vi "RenameEventNames.vi"(8 "Write":refnum<user-event>[](array[refnum]), 9 "Read":refnum<user-event>[](array[refnum]), 10 "State":refnum<user-event>[](array[refnum]), 11 "Error":refnum<user-event>[](array[refnum])) -> (0 "Write":refnum<user-event>[](array[refnum]), 1 "Read":refnum<user-event>[](array[refnum]), 2 "State":refnum<user-event>[](array[refnum]), 3 "Error":refnum<user-event>[](array[refnum]))   [LabVIEW 2016, in "lockin.lvclass"]
uses:
  lockin.lvclass
  DAQ/Typedefs/PublicEvents--DAQ.Read.ctl
  <vilib>/JKI/JKI SMO/SMO/Typedefs/SMOState --Enum.ctl
  DAQ/Typedefs/PublicEvents--DAQ.Write.ctl
  DAQ/DAQ.lvclass
  <vilib>/JKI/JKI SMO/SMO/SMO.lvclass
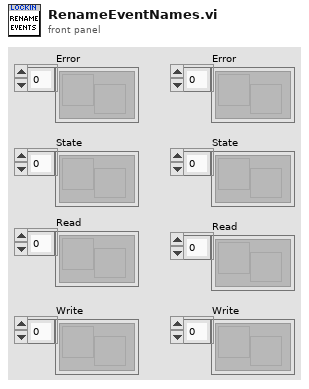
[diagram p1: front panel]
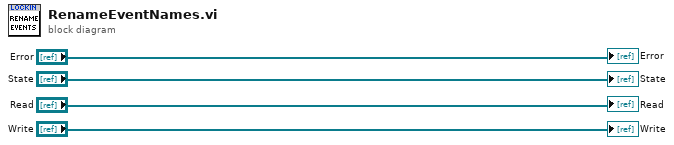
[diagram p0: block diagram]
diagram:
  "Read" <- "Read"
  "State" <- "State"
  "Error" <- "Error"
  "Write" <- "Write"
